vi "读取反控数据解析(子VI).vi"(6 "数据":string, 7 "命令编码CN":string) -> (0 "实时数据发送时间间隔/min":i32=1, 2 "设置超时时间/min":i32=1)   [LabVIEW 2016, in "数据传输系统.lvlib"]
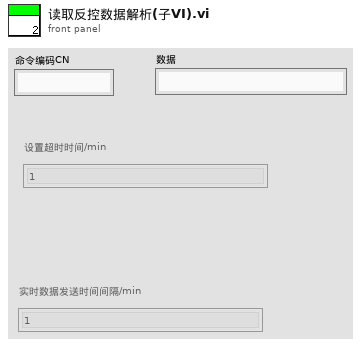
[diagram p1: front panel]
types:
  T1 = enum16{"初始化", "打开连接", "表格比对", "发送数据", "读取数据", "数据处理"}
  T2 = enum16{"CODMn", "CODCr", "氨氮", "总磷", "总氮", "数采仪"}
  T3 = cluster{"高锰酸盐":string, "化学需氧量":string, "氨氮":string, "总磷":string, "总氮":string, "数采仪":string, "高锰酸盐":bool, "化学需氧量":bool, "氨氮":bool, "总磷":bool, "总氮":bool, "数采仪":bool}
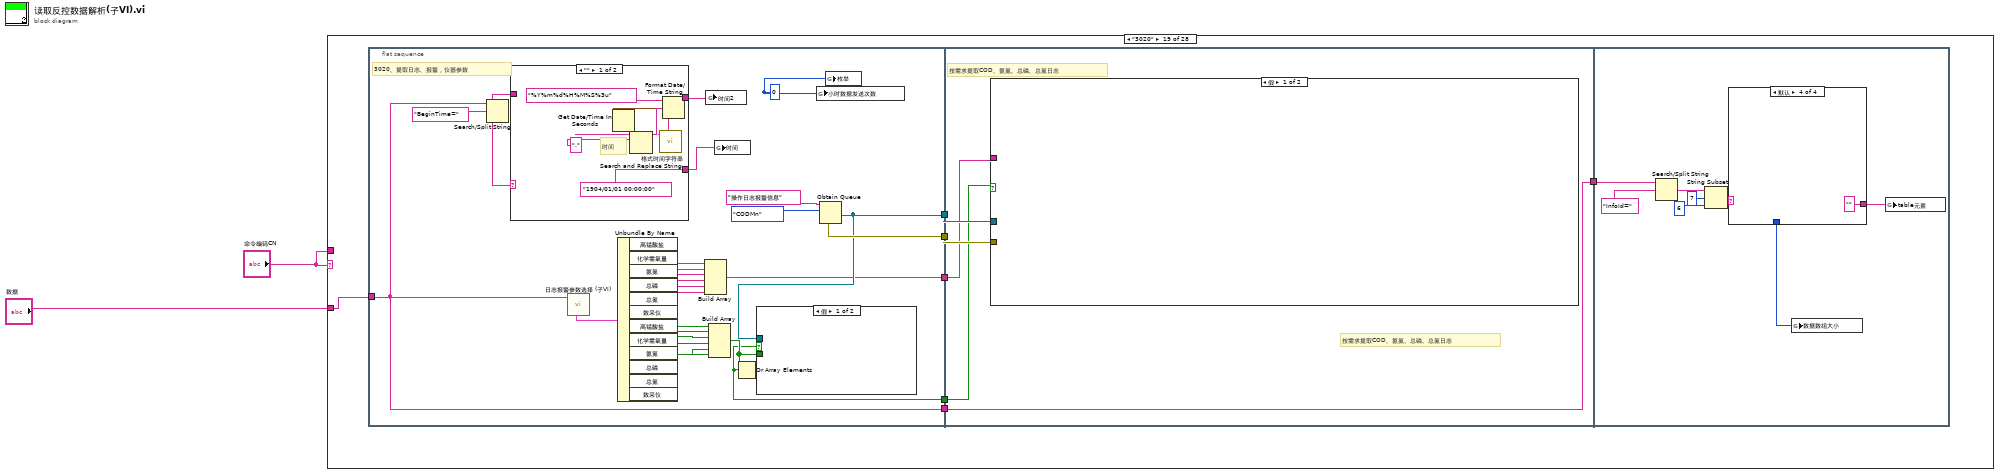
[diagram p0: block diagram]
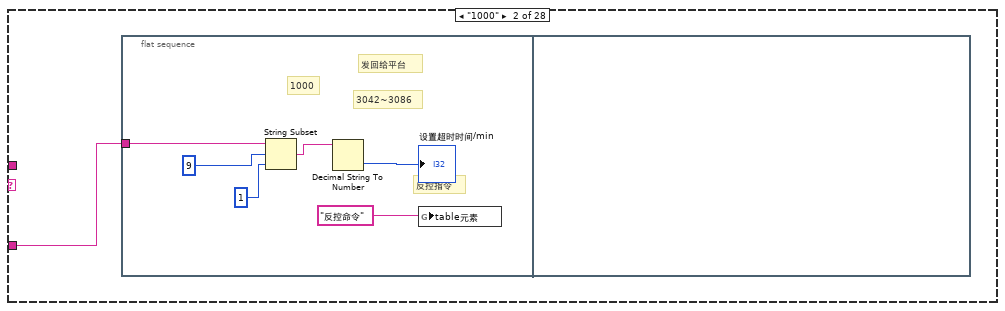
[diagram p3: hidden frame]
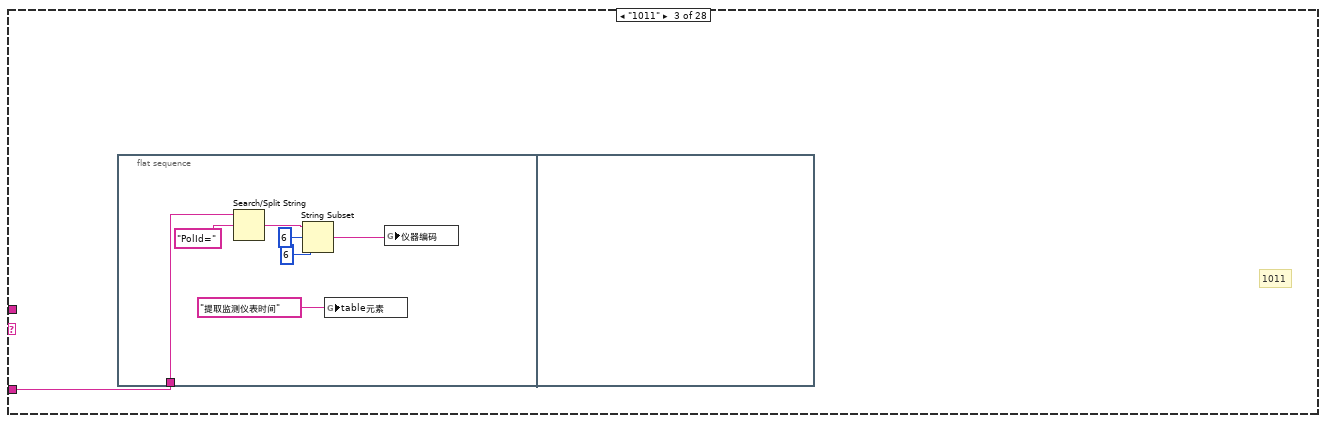
[diagram p4: hidden frame]
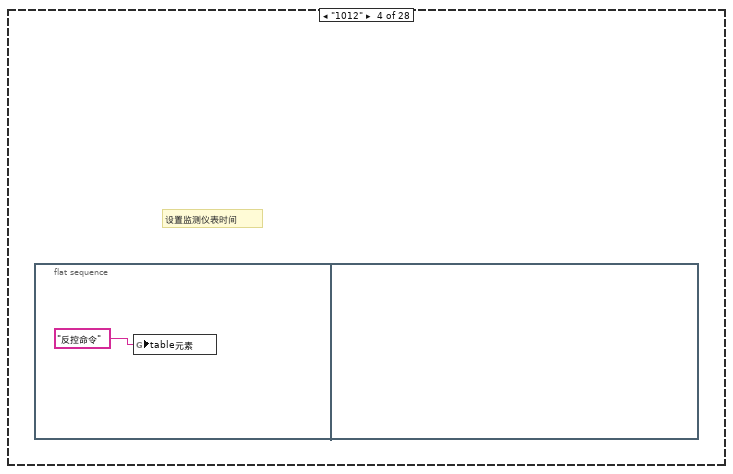
[diagram p5: hidden frame]
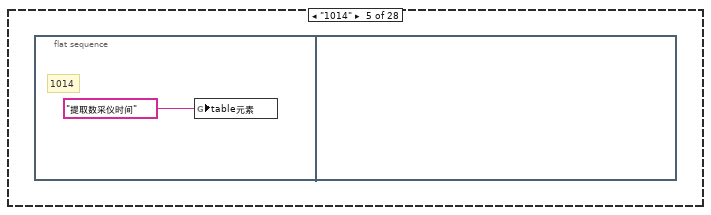
[diagram p6: hidden frame]
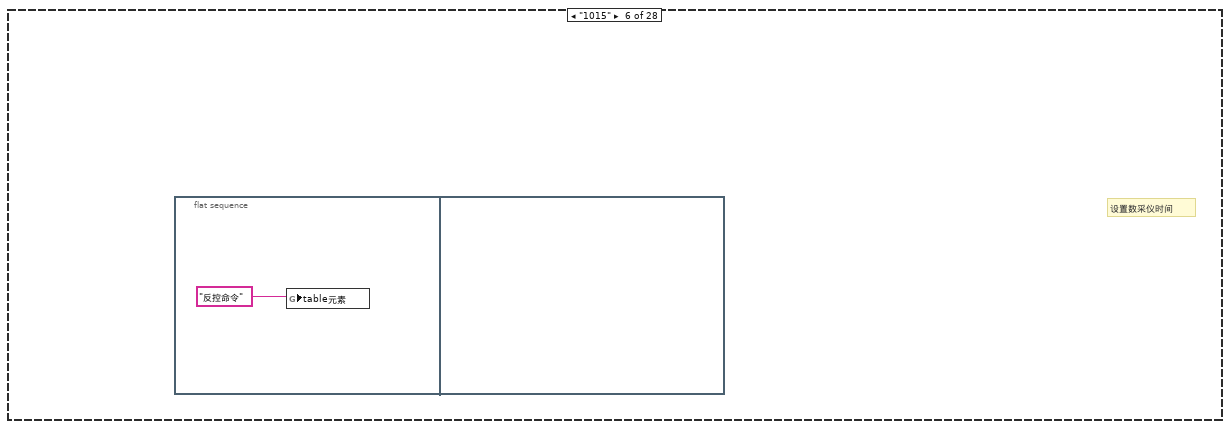
[diagram p7: hidden frame]
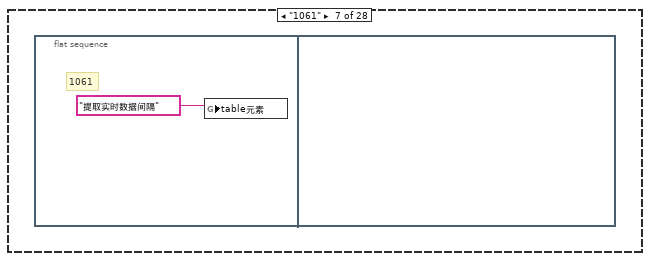
[diagram p8: hidden frame]
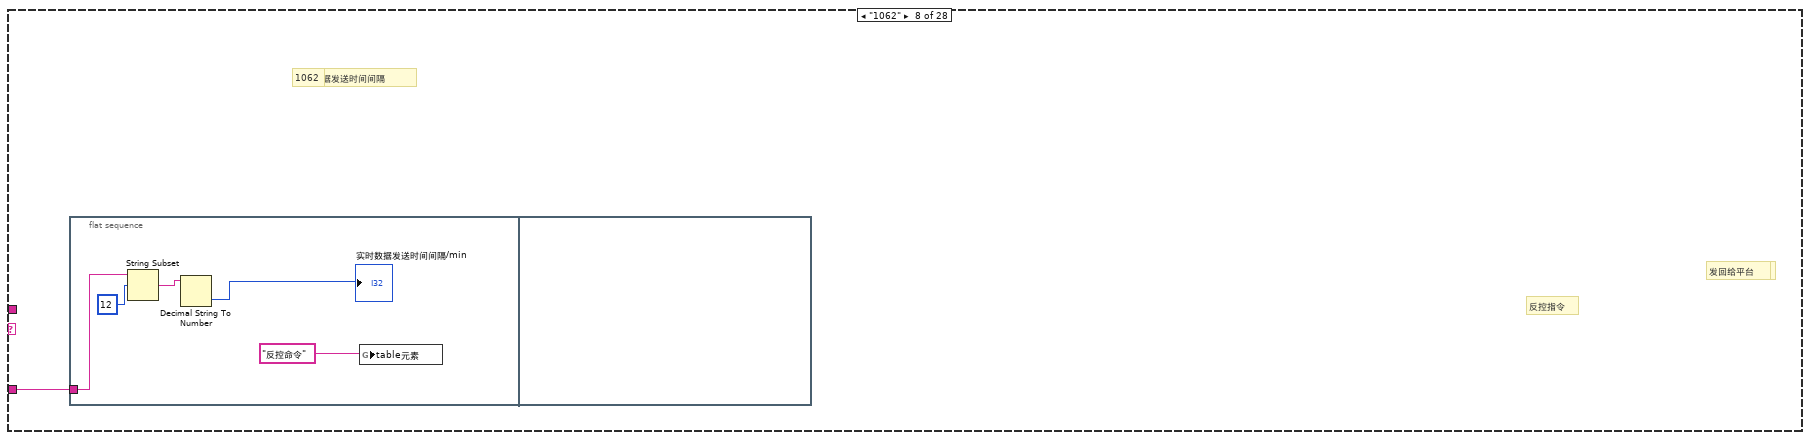
[diagram p9: hidden frame]
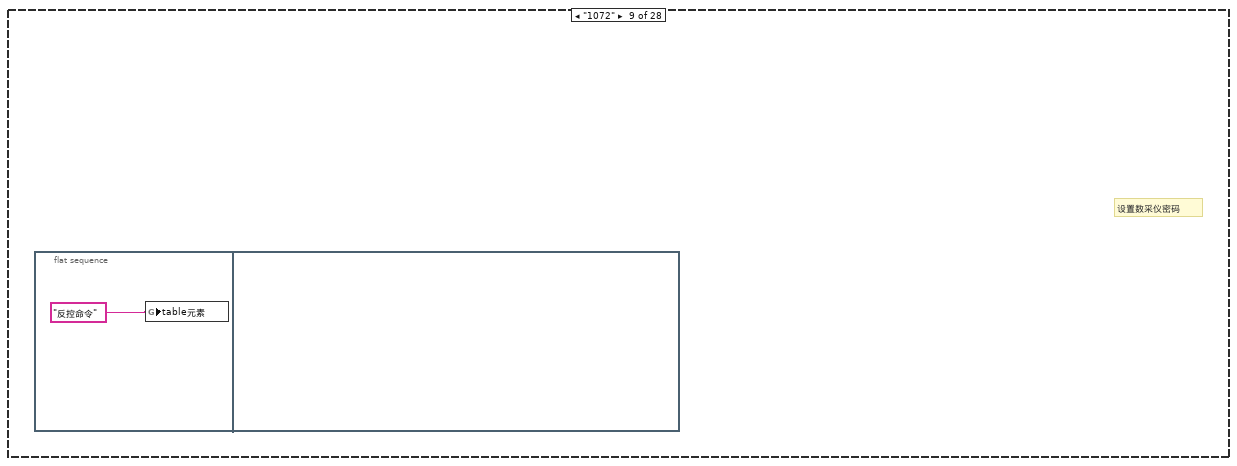
[diagram p10: hidden frame]
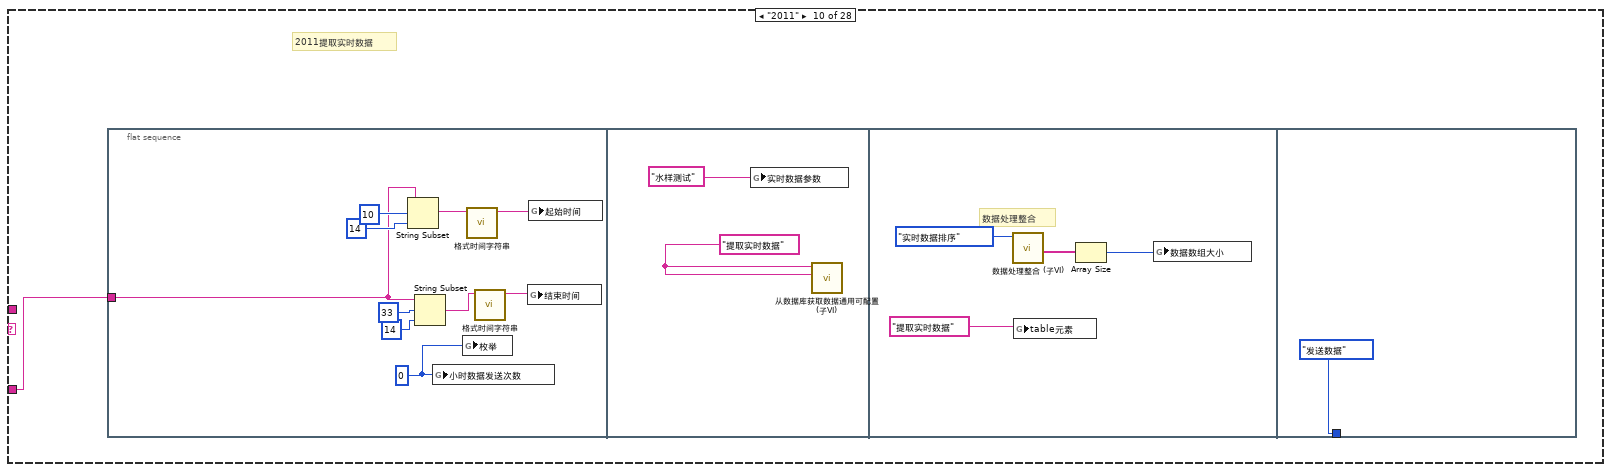
[diagram p11: hidden frame]
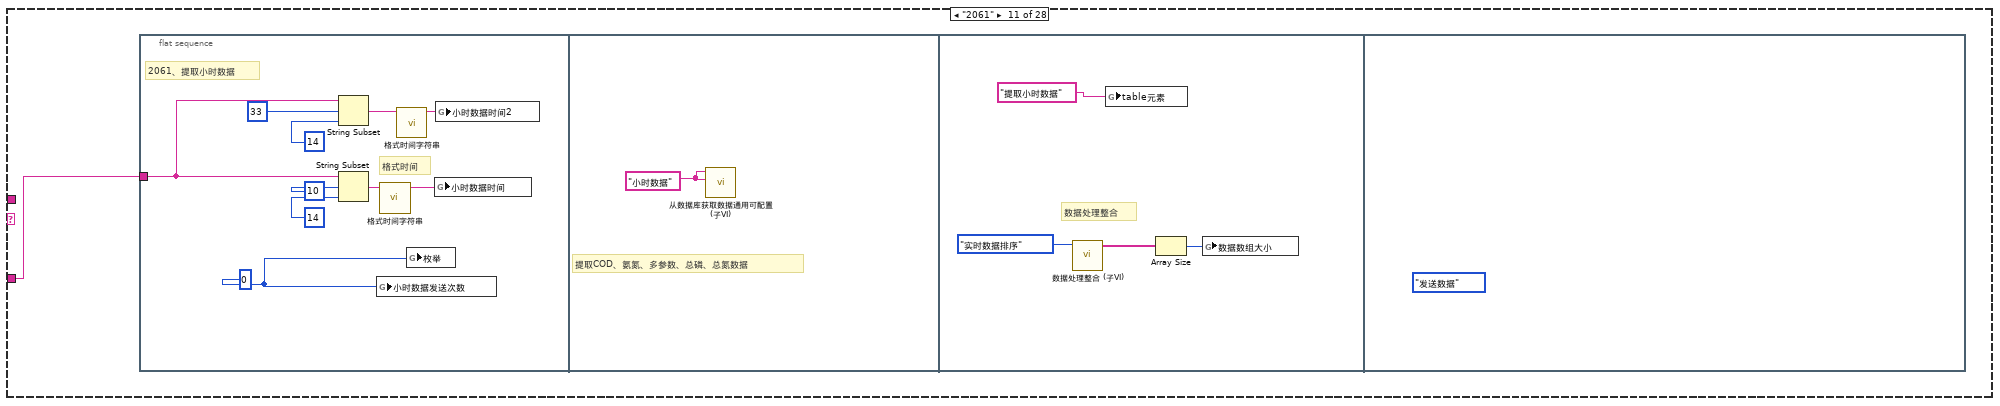
[diagram p12: hidden frame]
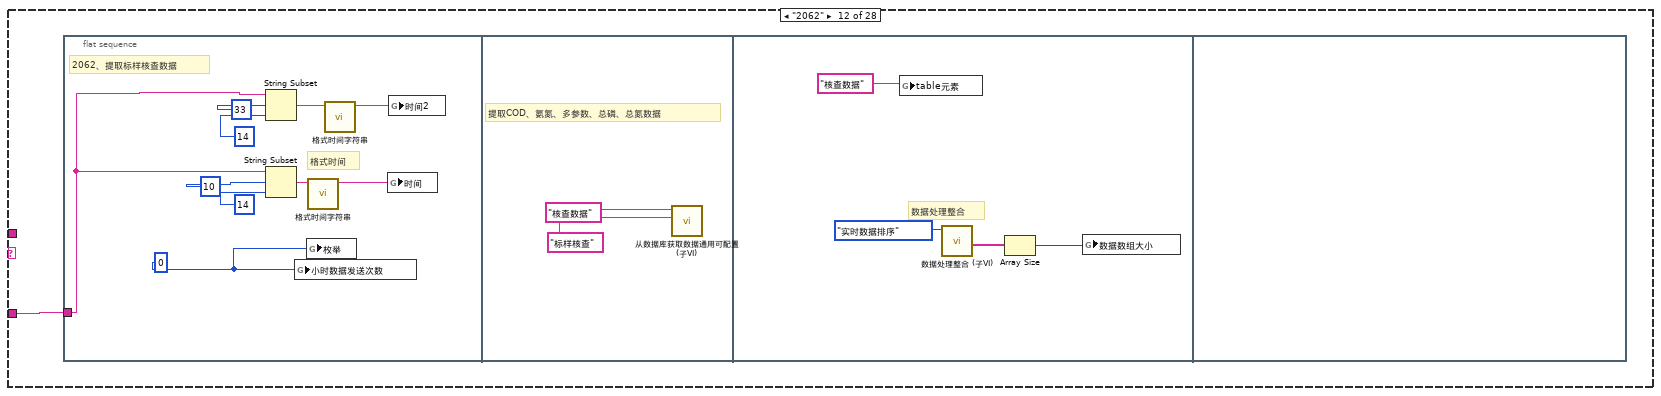
[diagram p13: hidden frame]
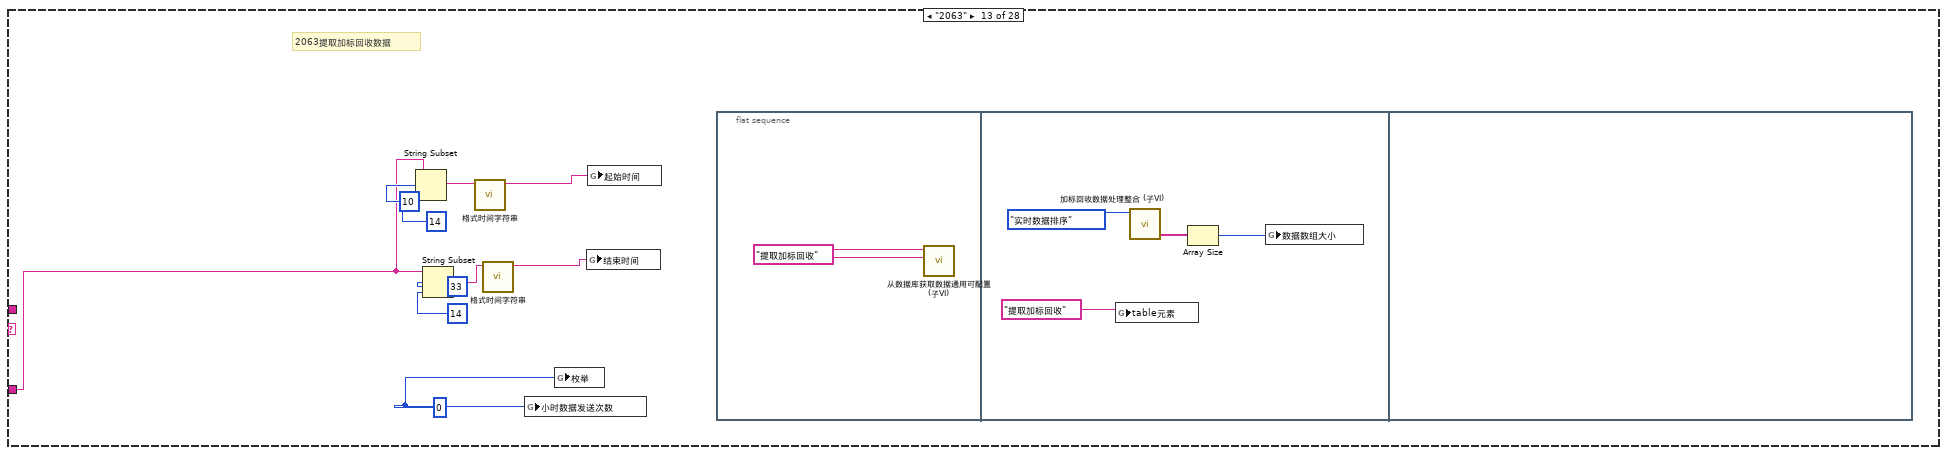
[diagram p14: hidden frame]
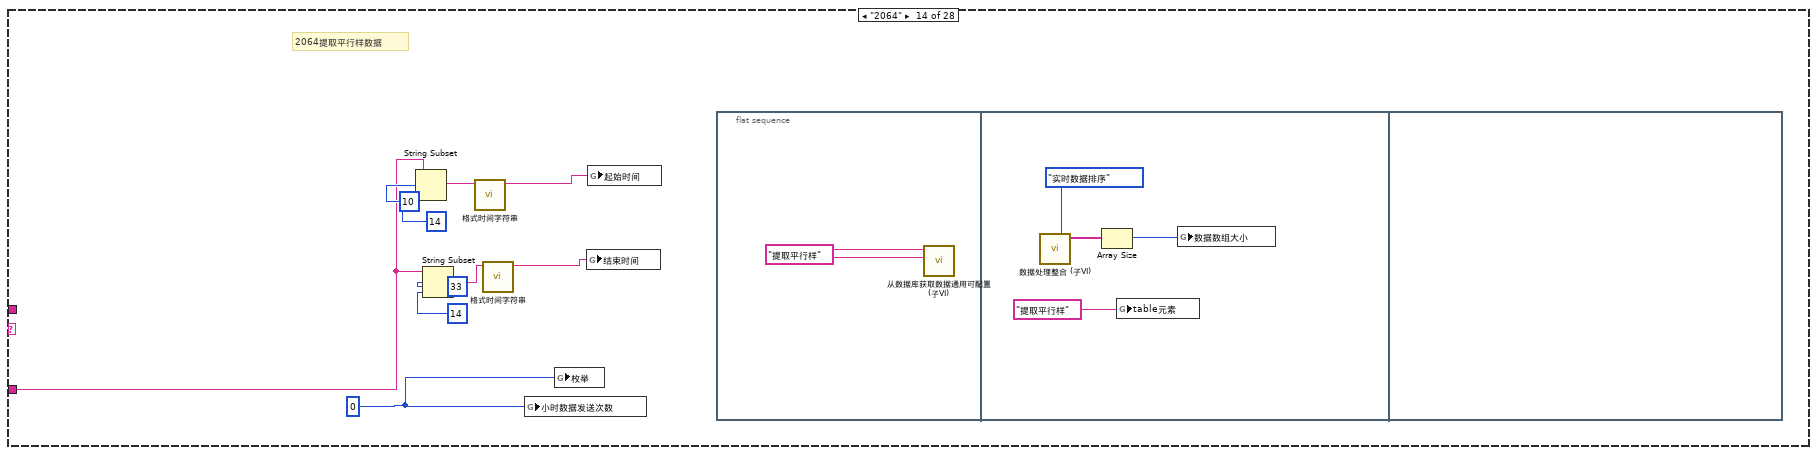
[diagram p15: hidden frame]
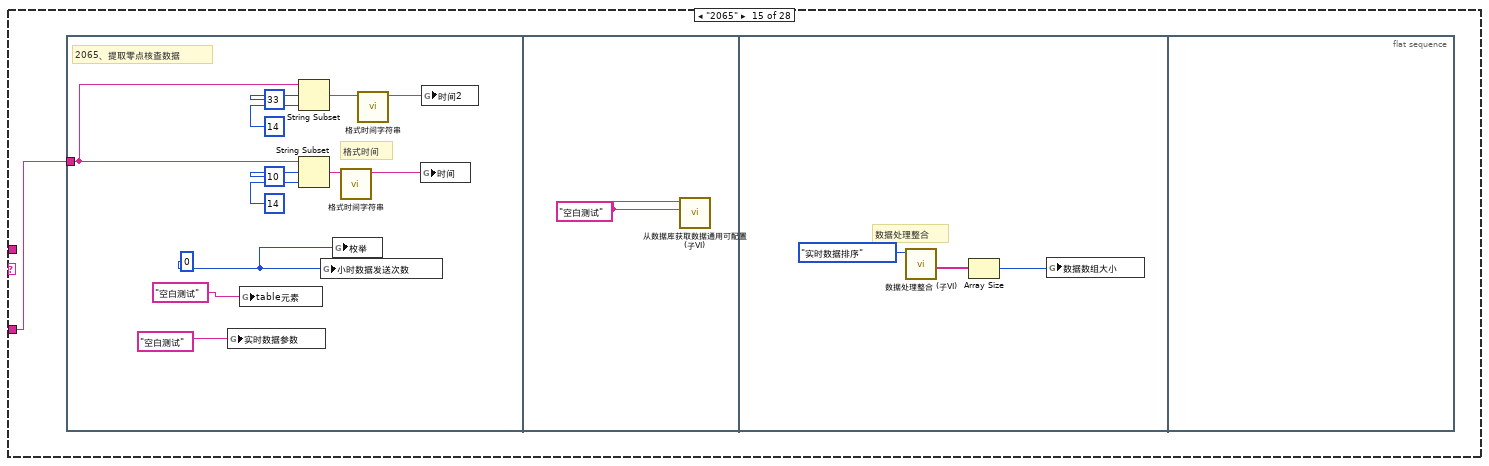
[diagram p16: hidden frame]
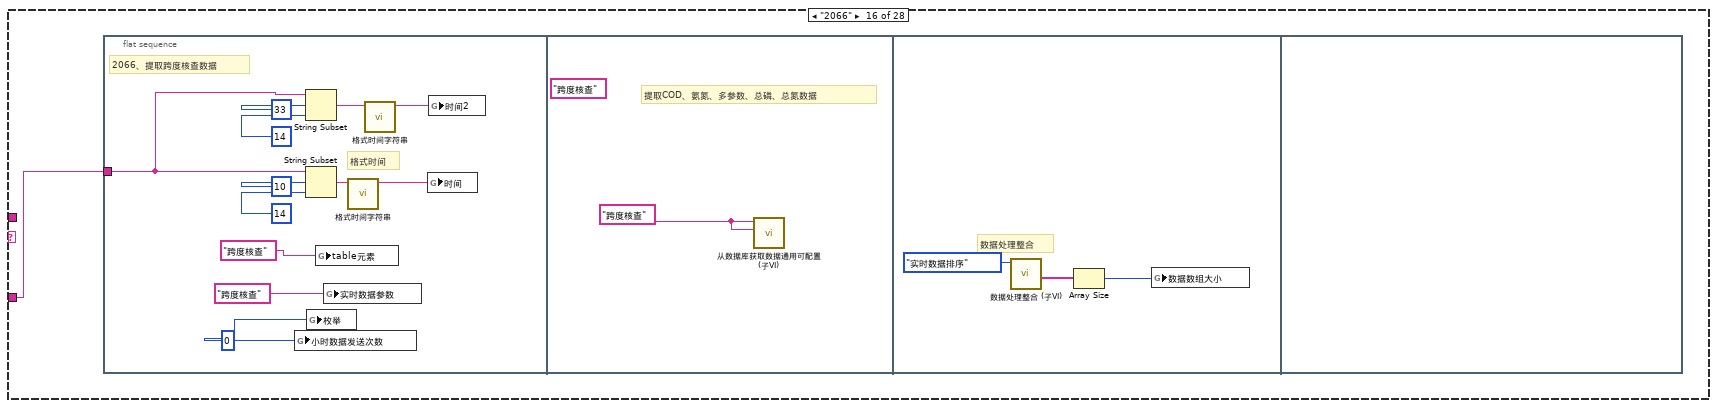
[diagram p17: hidden frame]
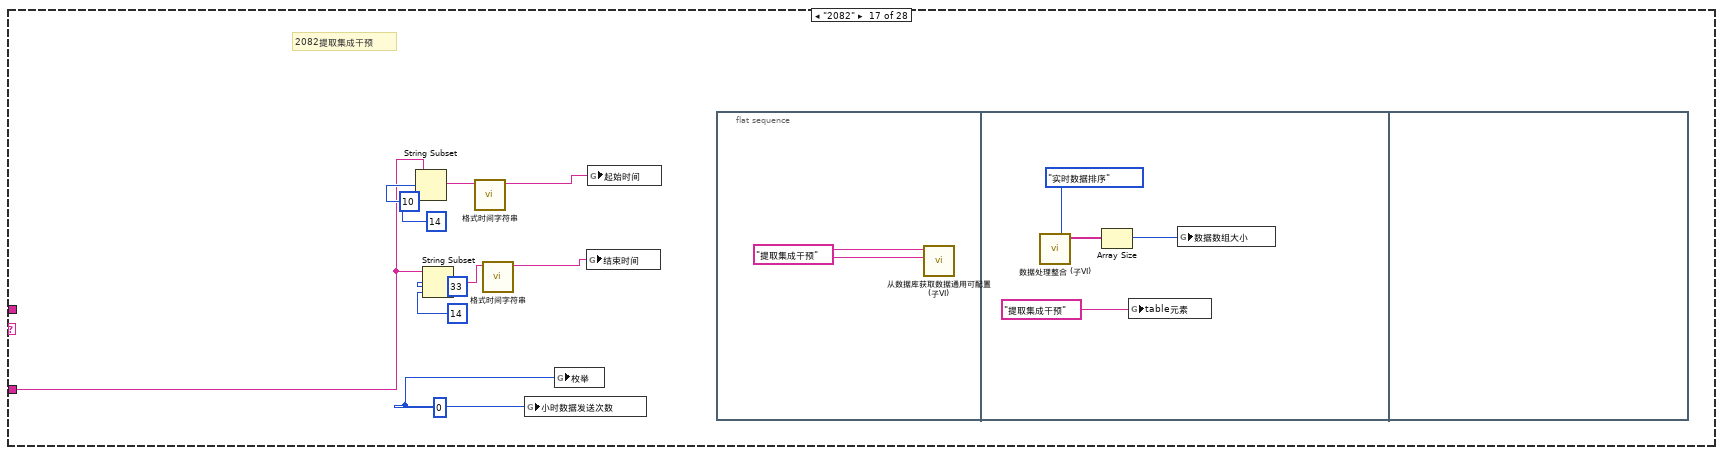
[diagram p18: hidden frame]
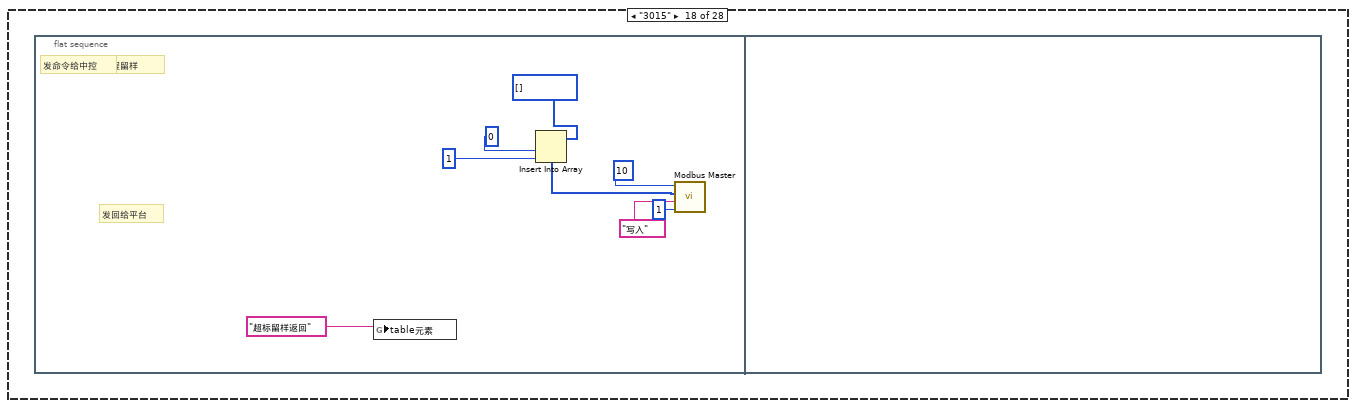
[diagram p19: hidden frame]
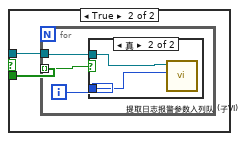
[diagram p20: hidden frame]
diagram:
  n1 = case shown="\"3020\"" "命令编码CN" {
    tunnel: "命令编码CN" -> [_ _ _ _ _ _ _ _ _ _ _ _ _ _ _ _ _ _ _ _ _ _ _ _ _ _ _ w353]
    tunnel: "数据" -> [_ w3 w10 _ _ _ _ w22 _ w29 w47 w63 w80 w95 w110 w127 w144 _ w169 _ _ _ w297 _ _ _ w337 w350]
    frame "", Default {
    }
    frame "1000" {
      n2 = flat-sequence {
        tunnel: w3 -> [w5]
        frame #0 {
          # "发回给平台"
          # "3042~3086"
          # "反控指令"
          # "1000"
          n3 = String Subset(string=w5, offset (0)=9 ("偏移量(0)"), length (rest)=1 ("长度（剩余）")) -> (substring=w7:string)
          n4 = Decimal String To Number(string=w7) -> (number=→"设置超时时间/min":i32)  [unwired: 2 in, 1 out]
          n5 = global write "全局1.vi" "table元素"("反控命令" ("新元素/子数组")) -> ()
        }
        frame #1 {
        }
      }
    }
    frame "1011" {
      # "1011"
      n6 = flat-sequence {
        tunnel: w10 -> [w12]
        frame #0 {
          n7 = Search/Split String(string=w12, search string/char (-)="PolId=" ("搜索字符串/字符(-)")) -> (match + rest of string=w16:string)  [unwired: 1 in, 2 out]
          n8 = String Subset(string=w16, offset (0)=6 ("偏移量(0)"), length (rest)=6 ("长度（剩余）")) -> (substring=w13:string)
          n9 = global write "全局1.vi" "table元素"("提取监测仪表时间") -> ()
          n10 = global write "全局 提取仪器参数.vi" "仪器编码"(w13) -> ()
        }
        frame #1 {
        }
      }
    }
    frame "1012" {
      # "设置监测仪表时间"
      n11 = flat-sequence {
        frame #0 {
          n12 = global write "全局1.vi" "table元素"("反控命令" ("新元素/子数组")) -> ()
        }
        frame #1 {
        }
      }
    }
    frame "1014" {
      n13 = flat-sequence {
        frame #0 {
          # "1014"
          n14 = global write "全局1.vi" "table元素"("提取数采仪时间") -> ()
        }
        frame #1 {
        }
      }
    }
    frame "1015" {
      # "设置数采仪时间"
      n15 = flat-sequence {
        frame #0 {
          n16 = global write "全局1.vi" "table元素"("反控命令" ("新元素/子数组")) -> ()
        }
        frame #1 {
        }
      }
    }
    frame "1061" {
      n17 = flat-sequence {
        frame #0 {
          # "1061"
          n18 = global write "全局1.vi" "table元素"("提取实时数据间隔") -> ()
        }
        frame #1 {
        }
      }
    }
    frame "1062" {
      # "发回给平台"
      # "反控指令"
      # "3042~3086"
      # "设置数据发送时间间隔"
      # "1062"
      n19 = flat-sequence {
        tunnel: w22 -> [w25]
        frame #0 {
          n20 = String Subset(string=w25, offset (0)=12 ("偏移量(0)")) -> (substring=w26:string)  [unwired: 1 in]
          n21 = Decimal String To Number(string=w26) -> (number=→"实时数据发送时间间隔/min":i32)  [unwired: 2 in, 1 out]
          n22 = global write "全局1.vi" "table元素"("反控命令" ("新元素/子数组")) -> ()
        }
        frame #1 {
        }
      }
    }
    frame "1072" {
      # "设置数采仪密码"
      n23 = flat-sequence {
        frame #0 {
          n24 = global write "全局1.vi" "table元素"("反控命令" ("新元素/子数组")) -> ()
        }
        frame #1 {
        }
      }
    }
    frame "2011" {
      # "2011提取实时数据"
      n25 = flat-sequence {
        tunnel: w29 -> [w30]
        tunnel: [T1."发送数据" ("元素")] -> _
        frame #0 {
          w35 = 0 ("数值")
          n26 = String Subset(string=w30, offset (0)=10 ("偏移量(0)"), length (rest)=14 ("长度（剩余）")) -> (substring=w38:string)
          n27 = String Subset(string=w30, offset (0)=33 ("偏移量(0)"), length (rest)=14 ("长度（剩余）")) -> (substring=w36:string)
          n28 = global write "全局 小时数据发送次数.vi" "小时数据发送次数"(w35) -> ()
          n29 = global write "全局1.vi" "枚举"(w35) -> ()
          n30 = call "格式时间字符串.vi"("字符串"=w38) -> ("连接的字符串"=w39:string)  [unwired: 10 in]
          n31 = call "格式时间字符串.vi"("字符串"=w36) -> ("连接的字符串"=w37:string)  [unwired: 10 in]
          n32 = global write "起始时间.vi" "结束时间"(w37) -> ()
          n33 = global write "起始时间.vi" "起始时间"(w39) -> ()
        }
        frame #1 {
          w40 = "提取实时数据" ("新元素/子数组")
          n34 = global write "全局 实时数据参数.vi" "实时数据参数"("水样测试") -> ()
          n35 = call "从数据库获取数据通用可配置(子VI).vi"("table输入"=w40, "列队名（唯一）"=w40) -> ()  [unwired: 8 in, 2 out]
        }
        frame #2 {
          # "数据处理整合"
          n36 = call "数据处理整合 (子VI).vi"("枚举"=enum16{"实时数据排序", "小时数据排序"}."实时数据排序") -> ("已排序的数组"=w44:string[])  [unwired: 10 in]
          n37 = global write "全局1.vi" "table元素"("提取实时数据" ("新元素/子数组")) -> ()
          n38 = Array Size(array=w44) -> (size(s)=w45:i32)
          n39 = global write "全局 数据数组大小.vi" "数据数组大小"(w45) -> ()
        }
        frame #3 {
        }
      }
    }
    frame "2061" {
      n40 = flat-sequence {
        tunnel: w47 -> [w48]
        frame #0 {
          w49 = 0 ("数值")
          # "格式时间"
          # "2061、提取小时数据"
          n41 = String Subset(string=w48, offset (0)=33 ("偏移量(0)"), length (rest)=14 ("长度（剩余）")) -> (substring=w51:string)
          n42 = String Subset(string=w48, offset (0)=10 ("偏移量(0)"), length (rest)=14 ("长度（剩余）")) -> (substring=w52:string)
          n43 = global write "全局 小时数据发送次数.vi" "小时数据发送次数"(w49) -> ()
          n44 = call "格式时间字符串.vi"("字符串"=w52) -> ("连接的字符串"=w53:string)  [unwired: 10 in]
          n45 = call "格式时间字符串.vi"("字符串"=w51) -> ("连接的字符串"=w50:string)  [unwired: 10 in]
          n46 = global write "全局1.vi" "枚举"(w49) -> ()
          n47 = global write "全局 水样时间.vi" "小时数据时间"(w53) -> ()
          n48 = global write "全局 时间2.vi" "小时数据时间2"(w50) -> ()
        }
        frame #1 {
          w58 = "小时数据" ("名称（未命名）")
          # "提取COD、氨氮、多参数、总磷、总氮数据"
          n49 = call "从数据库获取数据通用可配置(子VI).vi"("table输入"=w58, "列队名（唯一）"=w58) -> ()  [unwired: 8 in, 2 out]
        }
        frame #2 {
          # "数据处理整合"
          n50 = call "数据处理整合 (子VI).vi"("枚举"=enum16{"实时数据排序", "小时数据排序"}."实时数据排序") -> ("已排序的数组"=w62:string[])  [unwired: 10 in]
          n51 = global write "全局1.vi" "table元素"("提取小时数据" ("新元素/子数组")) -> ()
          n52 = Array Size(array=w62) -> (size(s)=w61:i32)
          n53 = global write "全局 数据数组大小.vi" "数据数组大小"(w61) -> ()
        }
        frame #3 {
          (unwired) T1."发送数据" ("元素")
        }
      }
    }
    frame "2062" {
      n54 = flat-sequence {
        tunnel: w63 -> [w64]
        frame #0 {
          w65 = 0 ("数值")
          # "格式时间"
          # "2062、提取标样核查数据"
          n55 = String Subset(string=w64, offset (0)=33 ("偏移量(0)"), length (rest)=14 ("长度（剩余）")) -> (substring=w67:string)
          n56 = String Subset(string=w64, offset (0)=10 ("偏移量(0)"), length (rest)=14 ("长度（剩余）")) -> (substring=w68:string)
          n57 = global write "全局 小时数据发送次数.vi" "小时数据发送次数"(w65) -> ()
          n58 = global write "全局1.vi" "枚举"(w65) -> ()
          n59 = call "格式时间字符串.vi"("字符串"=w68) -> ("连接的字符串"=w69:string)  [unwired: 10 in]
          n60 = call "格式时间字符串.vi"("字符串"=w67) -> ("连接的字符串"=w66:string)  [unwired: 10 in]
          n61 = global write "全局 水样时间.vi" "时间"(w69) -> ()
          n62 = global write "全局 时间2.vi" "时间2"(w66) -> ()
        }
        frame #1 {
          # "提取COD、氨氮、多参数、总磷、总氮数据"
          n63 = call "从数据库获取数据通用可配置(子VI).vi"("table输入"="标样核查" ("新元素/子数组"), "列队名（唯一）"="核查数据" ("新元素/子数组")) -> ()  [unwired: 8 in, 2 out]
        }
        frame #2 {
          # "数据处理整合"
          n64 = global write "全局1.vi" "table元素"("核查数据" ("新元素/子数组")) -> ()
          n65 = call "数据处理整合 (子VI).vi"("枚举"=enum16{"实时数据排序", "小时数据排序"}."实时数据排序") -> ("已排序的数组"=w78:string[])  [unwired: 10 in]
          n66 = Array Size(array=w78) -> (size(s)=w79:i32)
          n67 = global write "全局 数据数组大小.vi" "数据数组大小"(w79) -> ()
        }
        frame #3 {
        }
      }
    }
    frame "2063" {
      w85 = 0 ("数值")
      # "2063提取加标回收数据"
      n68 = String Subset(string=w80, offset (0)=10 ("偏移量(0)"), length (rest)=14 ("长度（剩余）")) -> (substring=w82:string)
      n69 = String Subset(string=w80, offset (0)=33 ("偏移量(0)"), length (rest)=14 ("长度（剩余）")) -> (substring=w84:string)
      n70 = call "格式时间字符串.vi"("字符串"=w82) -> ("连接的字符串"=w81:string)  [unwired: 10 in]
      n71 = call "格式时间字符串.vi"("字符串"=w84) -> ("连接的字符串"=w83:string)  [unwired: 10 in]
      n72 = global write "全局 小时数据发送次数.vi" "小时数据发送次数"(w85) -> ()
      n73 = global write "全局1.vi" "枚举"(w85) -> ()
      n74 = global write "起始时间.vi" "结束时间"(w83) -> ()
      n75 = global write "起始时间.vi" "起始时间"(w81) -> ()
      n76 = flat-sequence {
        frame #0 {
          w90 = "提取加标回收" ("新元素/子数组")
          n77 = call "从数据库获取数据通用可配置(子VI).vi"("table输入"=w90, "列队名（唯一）"=w90) -> ()  [unwired: 8 in, 2 out]
        }
        frame #1 {
          n78 = global write "全局1.vi" "table元素"("提取加标回收" ("新元素/子数组")) -> ()
          n79 = call "加标回收数据处理整合 (子VI).vi"("枚举"=enum16{"实时数据排序", "小时数据排序"}."实时数据排序") -> ("已排序的数组"=w92:string[])  [unwired: 10 in]
          n80 = Array Size(array=w92) -> (size(s)=w94:i32)
          n81 = global write "全局 数据数组大小.vi" "数据数组大小"(w94) -> ()
        }
        frame #2 {
        }
      }
    }
    frame "2064" {
      w100 = 0 ("数值")
      # "2064提取平行样数据"
      n82 = String Subset(string=w95, offset (0)=10 ("偏移量(0)"), length (rest)=14 ("长度（剩余）")) -> (substring=w97:string)
      n83 = String Subset(string=w95, offset (0)=33 ("偏移量(0)"), length (rest)=14 ("长度（剩余）")) -> (substring=w99:string)
      n84 = call "格式时间字符串.vi"("字符串"=w97) -> ("连接的字符串"=w96:string)  [unwired: 10 in]
      n85 = call "格式时间字符串.vi"("字符串"=w99) -> ("连接的字符串"=w98:string)  [unwired: 10 in]
      n86 = global write "全局 小时数据发送次数.vi" "小时数据发送次数"(w100) -> ()
      n87 = global write "全局1.vi" "枚举"(w100) -> ()
      n88 = global write "起始时间.vi" "结束时间"(w98) -> ()
      n89 = global write "起始时间.vi" "起始时间"(w96) -> ()
      n90 = flat-sequence {
        frame #0 {
          w105 = "提取平行样" ("新元素/子数组")
          n91 = call "从数据库获取数据通用可配置(子VI).vi"("table输入"=w105, "列队名（唯一）"=w105) -> ()  [unwired: 8 in, 2 out]
        }
        frame #1 {
          n92 = call "数据处理整合 (子VI).vi"("枚举"=enum16{"实时数据排序", "小时数据排序"}."实时数据排序") -> ("已排序的数组"=w109:string[])  [unwired: 10 in]
          n93 = Array Size(array=w109) -> (size(s)=w108:i32)
          n94 = global write "全局1.vi" "table元素"("提取平行样" ("新元素/子数组")) -> ()
          n95 = global write "全局 数据数组大小.vi" "数据数组大小"(w108) -> ()
        }
        frame #2 {
        }
      }
    }
    frame "2065" {
      n96 = flat-sequence {
        tunnel: w110 -> [w112]
        frame #0 {
          w113 = 0 ("数值")
          # "格式时间"
          # "2065、提取零点核查数据"
          n97 = global write "全局 实时数据参数.vi" "实时数据参数"("空白测试" ("新元素/子数组")) -> ()
          n98 = global write "全局1.vi" "table元素"("空白测试" ("新元素/子数组")) -> ()
          n99 = String Subset(string=w112, offset (0)=33 ("偏移量(0)"), length (rest)=14 ("长度（剩余）")) -> (substring=w116:string)
          n100 = String Subset(string=w112, offset (0)=10 ("偏移量(0)"), length (rest)=14 ("长度（剩余）")) -> (substring=w117:string)
          n101 = global write "全局 小时数据发送次数.vi" "小时数据发送次数"(w113) -> ()
          n102 = global write "全局1.vi" "枚举"(w113) -> ()
          n103 = call "格式时间字符串.vi"("字符串"=w117) -> ("连接的字符串"=w118:string)  [unwired: 10 in]
          n104 = call "格式时间字符串.vi"("字符串"=w116) -> ("连接的字符串"=w115:string)  [unwired: 10 in]
          n105 = global write "全局 水样时间.vi" "时间"(w118) -> ()
          n106 = global write "全局 时间2.vi" "时间2"(w115) -> ()
        }
        frame #1 {
          w123 = "空白测试" ("新元素/子数组")
          n107 = call "从数据库获取数据通用可配置(子VI).vi"("table输入"=w123, "列队名（唯一）"=w123) -> ()  [unwired: 8 in, 2 out]
        }
        frame #2 {
          # "数据处理整合"
          n108 = call "数据处理整合 (子VI).vi"("枚举"=enum16{"实时数据排序", "小时数据排序"}."实时数据排序") -> ("已排序的数组"=w125:string[])  [unwired: 10 in]
          n109 = Array Size(array=w125) -> (size(s)=w126:i32)
          n110 = global write "全局 数据数组大小.vi" "数据数组大小"(w126) -> ()
        }
        frame #3 {
        }
      }
    }
    frame "2066" {
      n111 = flat-sequence {
        tunnel: w127 -> [w129]
        frame #0 {
          w130 = 0 ("数值")
          # "格式时间"
          # "2066、提取跨度核查数据"
          n112 = global write "全局 小时数据发送次数.vi" "小时数据发送次数"(w130) -> ()
          n113 = String Subset(string=w129, offset (0)=33 ("偏移量(0)"), length (rest)=14 ("长度（剩余）")) -> (substring=w133:string)
          n114 = String Subset(string=w129, offset (0)=10 ("偏移量(0)"), length (rest)=14 ("长度（剩余）")) -> (substring=w134:string)
          n115 = global write "全局1.vi" "枚举"(w130) -> ()
          n116 = global write "全局1.vi" "table元素"("跨度核查" ("新元素/子数组")) -> ()
          n117 = global write "全局 实时数据参数.vi" "实时数据参数"("跨度核查" ("新元素/子数组")) -> ()
          n118 = call "格式时间字符串.vi"("字符串"=w134) -> ("连接的字符串"=w135:string)  [unwired: 10 in]
          n119 = call "格式时间字符串.vi"("字符串"=w133) -> ("连接的字符串"=w132:string)  [unwired: 10 in]
          n120 = global write "全局 水样时间.vi" "时间"(w135) -> ()
          n121 = global write "全局 时间2.vi" "时间2"(w132) -> ()
        }
        frame #1 {
          w140 = "跨度核查" ("新元素/子数组")
          (unwired) "跨度核查" ("名称（未命名）")
          # "提取COD、氨氮、多参数、总磷、总氮数据"
          n122 = call "从数据库获取数据通用可配置(子VI).vi"("table输入"=w140, "列队名（唯一）"=w140) -> ()  [unwired: 8 in, 2 out]
        }
        frame #2 {
          # "数据处理整合"
          n123 = call "数据处理整合 (子VI).vi"("枚举"=enum16{"实时数据排序", "小时数据排序"}."实时数据排序") -> ("已排序的数组"=w143:string[])  [unwired: 10 in]
          n124 = Array Size(array=w143) -> (size(s)=w142:i32)
          n125 = global write "全局 数据数组大小.vi" "数据数组大小"(w142) -> ()
        }
        frame #3 {
        }
      }
    }
    frame "2082" {
      w149 = 0 ("数值")
      # "2082提取集成干预"
      n126 = String Subset(string=w144, offset (0)=10 ("偏移量(0)"), length (rest)=14 ("长度（剩余）")) -> (substring=w146:string)
      n127 = String Subset(string=w144, offset (0)=33 ("偏移量(0)"), length (rest)=14 ("长度（剩余）")) -> (substring=w148:string)
      n128 = call "格式时间字符串.vi"("字符串"=w146) -> ("连接的字符串"=w145:string)  [unwired: 10 in]
      n129 = call "格式时间字符串.vi"("字符串"=w148) -> ("连接的字符串"=w147:string)  [unwired: 10 in]
      n130 = global write "全局 小时数据发送次数.vi" "小时数据发送次数"(w149) -> ()
      n131 = global write "全局1.vi" "枚举"(w149) -> ()
      n132 = global write "起始时间.vi" "结束时间"(w147) -> ()
      n133 = global write "起始时间.vi" "起始时间"(w145) -> ()
      n134 = flat-sequence {
        frame #0 {
          w154 = "提取集成干预" ("新元素/子数组")
          n135 = call "从数据库获取数据通用可配置(子VI).vi"("table输入"=w154, "列队名（唯一）"=w154) -> ()  [unwired: 8 in, 2 out]
        }
        frame #1 {
          n136 = call "数据处理整合 (子VI).vi"("枚举"=enum16{"实时数据排序", "小时数据排序"}."实时数据排序") -> ("已排序的数组"=w158:string[])  [unwired: 10 in]
          n137 = Array Size(array=w158) -> (size(s)=w157:i32)
          n138 = global write "全局1.vi" "table元素"("提取集成干预" ("新元素/子数组")) -> ()
          n139 = global write "全局 数据数组大小.vi" "数据数组大小"(w157) -> ()
        }
        frame #2 {
        }
      }
    }
    frame "3015" {
      n140 = flat-sequence {
        frame #0 {
          # "发命令给中控"
          # "发回给平台"
          # "3015、手动远程留样"
          n141 = global write "全局1.vi" "table元素"("超标留样返回" ("新元素/子数组")) -> ()
          n142 = Insert Into Array(array=u16[] [] ("holding register values"), index=0 ("索引"), new element=u16 1 ("新元素/子数组")) -> (w162:u16[])
          n143 = call "Modbus Master.vi"("Unit ID"=u8 1, "读取写入选择"="写入", "holding register values"=w162, "starting address"=u16 10) -> ()  [unwired: 6 in, 2 out]
        }
        frame #1 {
        }
      }
    }
    frame "3020" {
      n144 = flat-sequence {
        tunnel: [w178] -> w173
        tunnel: [w179] -> w172
        tunnel: [w177] -> w171
        tunnel: [w175] -> w170
        tunnel: w169 -> [w174]
        tunnel: [w174] -> w167
        tunnel: w173 -> [w227]
        tunnel: w172 -> [w226]
        tunnel: w171 -> [w225]
        tunnel: w170 -> [w224]
        tunnel: [w223] -> w168
        tunnel: w167 -> [w223]
        tunnel: w168 -> [w275]
        frame #0 {
          w197 = 0 ("数值")
          # "3020、提取日志、报警，仪器参数"
          n145 = Search/Split String(string=w174, search string/char (-)="BeginTime=" ("搜索字符串")) -> (match + rest of string=w196:string)  [unwired: 1 in, 2 out]
          n146 = case shown="\"\"" w196 {
            tunnel: ["1904/01/01 00:00:00" w220] -> w199
            tunnel: w196 -> [_ w214]
            tunnel: [w207 w215] -> w195
            frame "" {
              # "时间"
              n147 = Get Date/Time In Seconds() -> (seconds since 1Jan1904=w208:timestamp)
              n148 = Format Date/Time String(time format string (%c)="%Y%m%d%H%M%S%3u" ("时间格式字符串(%c)"), seconds (now)=w208) -> (date/time string=w212:string)  [unwired: 1 in]
              n149 = Search and Replace String(input string=w212, search string="." ("搜索字符串")) -> (result string=w211:string)  [unwired: 6 in, 3 out]
              n150 = call "格式时间字符串.vi"("字符串"=w211) -> ("连接的字符串"=w207:string)  [unwired: 10 in]
            }
            frame "真", Default {
              # "格式时间"
              n151 = String Subset(string=w214, offset (0)=33 ("偏移量(0)"), length (rest)=14 ("长度（剩余）")) -> (substring=w218:string)
              n152 = String Subset(string=w214, offset (0)=10 ("偏移量(0)"), length (rest)=14 ("长度（剩余）")) -> (substring=w219:string)
              n153 = call "格式时间字符串.vi"("字符串"=w218) -> ("连接的字符串"=w215:string)  [unwired: 10 in]
              n154 = call "格式时间字符串.vi"("字符串"=w219) -> ("连接的字符串"=w220:string)  [unwired: 10 in]
            }
          }
          n155 = call "日志报警参数选择 (子VI).vi"("String输入"=w174) -> ("输出簇"=w182:T3)  [unwired: 9 in, 1 out]
          n156 = Unbundle By Name(w182) -> ("高锰酸盐"=w189:string, "化学需氧量"=w190:string, "氨氮"=w191:string, "总磷"=w192:string, "总氮"=w193:string, "数采仪"=w194:string, "高锰酸盐"=w183:bool, "化学需氧量"=w184:bool, "氨氮"=w185:bool, "总磷"=w186:bool, "总氮"=w187:bool, "数采仪"=w188:bool)
          n157 = Build Array(w189, w190, w191, w192, w193, w194) -> (w177:string[])
          n158 = global write "全局 时间2.vi" "时间2"(w195) -> ()
          n159 = Build Array(w183, w184, w185, w186, w187, w188) -> (w176:bool[])
          n160 = global write "全局 水样时间.vi" "时间"(w199) -> ()
          n161 = Or Array Elements(Boolean array=w176) -> (logical OR=w175:bool)
          n162 = global write "全局 小时数据发送次数.vi" "小时数据发送次数"(w197) -> ()
          n163 = Obtain Queue(name (unnamed)="操作日志报警信息" ("名称（未命名）"), element data type=T2."CODMn") -> (queue out=w178:refnum<queue>, error out=w179:errorcluster)  [unwired: 3 in, 1 out]
          n164 = case shown="假" w175 {
            tunnel: w178 -> [_ w201]
            tunnel: w176 -> [_ w200]
            frame False {
            }
            frame True {
              n165 = for {
                tunnel: w200 -> [w203] mode=indexing
                tunnel: w201 -> [w202]
                i -> [w204]
                n166 = case shown="真" w203 {
                  tunnel: w204 -> [_ w206]
                  tunnel: w202 -> [_ w205]
                  frame False {
                  }
                  frame True {
                    n167 = call "提取日志报警参数入列队 (子VI).vi"("枚举"=w206, "queue in"=w205) -> ()  [unwired: 10 in]
                  }
                }
              }
            }
          }
          n168 = global write "全局1.vi" "枚举"(w197) -> ()
        }
        frame #1 {
          # "按需求提取COD、氨氮、总磷、总氮日志"
          # "按需求提取COD、氨氮、总磷、总氮日志"
          n169 = case shown="假" w224 {
            tunnel: w226 -> [_ w230]
            tunnel: w227 -> [_ w229]
            tunnel: w225 -> [_ w228]
            frame False {
            }
            frame True {
              n170 = while {
                shift-right: [w244] -> _
                shift-left: w229 -> [w245]
                tunnel: w230 -> [w243]
                tunnel: w228 -> [w238]
                stop <- w240 stop-if-true
                n171 = Dequeue Element(queue=w245, error in (no error)=w243) -> (queue out=w242:refnum<queue>, element=w237:T2)  [unwired: 1 in, 2 out]
                n172 = Index Array(array=w238) -> (element #1=w236:string, element #2=w235:string, element #3=w234:string, element #4=w233:string, element #5=w232:string, element #6=w231:string)  [unwired: 6 in]
                n173 = case shown="\"CODMn\"" w237 {
                  tunnel: w242 -> [w250 _ w259 w264 w268 w273]
                  tunnel: [w250 _ w259 w264 w268 w273] -> w244
                  tunnel: w236 -> [w247 _ _ _ _ _]
                  tunnel: w235 -> [_ w252 _ _ _ _]
                  tunnel: w234 -> [_ _ w256 _ _ _]
                  tunnel: w233 -> [_ _ _ w261 _ _]
                  tunnel: w232 -> [_ _ _ _ w266 _]
                  tunnel: w231 -> [_ _ _ _ _ w270]
                  frame "CODMn" {
                    w246 = string[][] [] ("氨氮")
                    n174 = call "数据表比对.vi"("仪器日志参数"="CODMn" ("元素"), "table输入"=w247) -> ("待发送数据"=w248:string[][])  [unwired: 7 in, 2 out]
                    n175 = global write "全局 所有参数.vi" "CODMn"(w248) -> ()
                    n176 = global write "全局 所有参数.vi" "总氮"(w246) -> ()
                    n177 = global write "全局 所有参数.vi" "CODCr"(w246) -> ()
                    n178 = global write "全局 所有参数.vi" "总磷"(w246) -> ()
                    n179 = global write "全局 所有参数.vi" "氨氮"(w246) -> ()
                  }
                  frame "CODCr" {
                    w251 = string[][] [] ("氨氮")
                    n180 = call "数据表比对.vi"("仪器日志参数"="CODCr" ("元素"), "table输入"=w252) -> ("待发送数据"=w253:string[][])  [unwired: 7 in, 2 out]
                    n181 = global write "全局 所有参数.vi" "CODCr"(w253) -> ()
                    n182 = global write "全局 所有参数.vi" "CODMn"(w251) -> ()
                    n183 = global write "全局 所有参数.vi" "总氮"(w251) -> ()
                    n184 = global write "全局 所有参数.vi" "总磷"(w251) -> ()
                    n185 = global write "全局 所有参数.vi" "氨氮"(w251) -> ()
                  }
                  frame "氨氮" {
                    w255 = string[][] [] ("氨氮")
                    n186 = call "数据表比对.vi"("仪器日志参数"="氨氮" ("元素"), "table输入"=w256) -> ("待发送数据"=w257:string[][])  [unwired: 7 in, 2 out]
                    n187 = global write "全局 所有参数.vi" "氨氮"(w257) -> ()
                    n188 = global write "全局 所有参数.vi" "CODMn"(w255) -> ()
                    n189 = global write "全局 所有参数.vi" "总氮"(w255) -> ()
                    n190 = global write "全局 所有参数.vi" "CODCr"(w255) -> ()
                    n191 = global write "全局 所有参数.vi" "总磷"(w255) -> ()
                  }
                  frame "总磷" {
                    w260 = string[][] [] ("氨氮")
                    n192 = call "数据表比对.vi"("仪器日志参数"="总磷" ("元素"), "table输入"=w261) -> ("待发送数据"=w262:string[][])  [unwired: 7 in, 2 out]
                    n193 = global write "全局 所有参数.vi" "总磷"(w262) -> ()
                    n194 = global write "全局 所有参数.vi" "CODMn"(w260) -> ()
                    n195 = global write "全局 所有参数.vi" "总氮"(w260) -> ()
                    n196 = global write "全局 所有参数.vi" "CODCr"(w260) -> ()
                    n197 = global write "全局 所有参数.vi" "氨氮"(w260) -> ()
                  }
                  frame "总氮" {
                    w265 = string[][] [] ("氨氮")
                    n198 = call "数据表比对.vi"("仪器日志参数"="总氮" ("元素"), "table输入"=w266) -> ("待发送数据"=w267:string[][])  [unwired: 7 in, 2 out]
                    n199 = global write "全局 所有参数.vi" "总氮"(w267) -> ()
                    n200 = global write "全局 所有参数.vi" "CODMn"(w265) -> ()
                    n201 = global write "全局 所有参数.vi" "氨氮"(w265) -> ()
                    n202 = global write "全局 所有参数.vi" "CODCr"(w265) -> ()
                    n203 = global write "全局 所有参数.vi" "总磷"(w265) -> ()
                  }
                  frame "数采仪" {
                    n204 = call "数据表比对.vi"("仪器日志参数"="系统" ("元素"), "table输入"=w270) -> ("待发送数据"=w271:string[][])  [unwired: 7 in, 2 out]
                    n205 = global write "全局 所有参数.vi" "DO"(w271) -> ()
                  }
                }
                n206 = Get Queue Status(queue=w242) -> (# elements in queue=w241:i32)  [unwired: 2 in, 7 out]
                n207 = Wait (ms)(milliseconds to wait=u32 300 ("等待时间（毫秒）")) -> ()  [unwired: 1 out]
                n208 = Equal To 0?(x=w241) -> (x = 0?=w240:bool)
              }
            }
          }
        }
        frame #2 {
          n209 = Search/Split String(string=w275, search string/char (-)="InfoId=" ("搜索字符串/字符(-)")) -> (match + rest of string=w280:string)  [unwired: 1 in, 2 out]
          n210 = String Subset(string=w280, offset (0)=7 ("偏移量(0)"), length (rest)=6 ("长度（剩余）")) -> (substring=w277:string)
          n211 = case shown="默认" w277 {
            selector: w277 -> [_ w286 _ _]
            tunnel: ["操作日志" ("名称（未命名）") "提取仪器参数" ("名称（未命名）") "报警信息" ("名称（未命名）") "" ("名称（未命名）")] -> w274
            tunnel: [w282 1 ("数据数组大小") w289 _] -> w276
            frame "i11001", "i21001" {
              # "数据处理整合"
              # "i11001日志"
              n212 = call "数据处理整合 (子VI).vi"("枚举"=enum16{"实时数据排序", "小时数据排序"}."实时数据排序") -> ("已排序的数组"=w283:string[])  [unwired: 10 in]
              n213 = Array Size(array=w283) -> (size(s)=w282:i32)
            }
            frame "i13001", "i13002", "i13003", "i13004", "i13005", "i13006", "i13007", "i13008", "i13009", "i13010", "i13011", "i13012", "i13013" {
              n214 = global write "全局 提取仪器参数.vi" "参数编码"(w286) -> ()
              n215 = call "数据处理直接插入整合 (子VI).vi"() -> ()  [unwired: 12 in]
            }
            frame "i12001" {
              # "数据处理整合"
              # "i12001状态"
              n216 = call "数据处理整合 (子VI).vi"("枚举"=enum16{"实时数据排序", "小时数据排序"}."实时数据排序") -> ("已排序的数组"=w290:string[])  [unwired: 10 in]
              n217 = Array Size(array=w290) -> (size(s)=w289:i32)
            }
            frame Default {
            }
          }
          n218 = global write "全局 数据数组大小.vi" "数据数组大小"(w276) -> ()
          n219 = global write "全局1.vi" "table元素"(w274) -> ()
        }
      }
    }
    frame "3021" {
      n220 = flat-sequence {
        frame #0 {
          # "设置仪表参数"
          n221 = global write "全局1.vi" "table元素"("反控命令" ("新元素/子数组")) -> ()
        }
        frame #1 {
        }
      }
    }
    frame "3040" {
      # "提取现场系统信息（3040）"
      n222 = flat-sequence {
        frame #0 {
          n223 = global write "全局1.vi" "table元素"("提取现场系统信息" ("新元素/子数组")) -> ()
        }
        frame #1 {
        }
      }
    }
    frame "3041" {
      # "提取现场经纬度及环境信息（3041）"
      n224 = flat-sequence {
        frame #0 {
          n225 = call "获取环境参数 (子VI).vi"() -> ()  [unwired: 12 in]
          n226 = global write "全局1.vi" "table元素"("提取经纬度环境信息" ("新元素/子数组")) -> ()
        }
        frame #1 {
        }
      }
    }
    frame "3042" {
      n227 = flat-sequence {
        tunnel: w297 -> [w299]
        frame #0 {
          # "反控指令"
          # "反控指令\n切换运行模式"
          # "发命令给中控"
          # "0维护，1常规，2应急，3质控"
          n228 = Search/Split String(string=w299, search string/char (-)="RunMode" ("搜索字符串/字符(-)")) -> (match + rest of string=w310:string)  [unwired: 1 in, 2 out]
          n229 = String Subset(string=w310, offset (0)=8 ("偏移量(0)"), length (rest)=1 ("长度（剩余）")) -> (substring=w307:string)
          n230 = case shown="\"2\"" w307 {
            tunnel: [u16 0 ("新元素/子数组") u16 1 ("新元素/子数组") u16 2 ("新元素/子数组") u16 3 ("新元素/子数组")] -> w303
            frame "0", Default {
            }
            frame "1" {
            }
            frame "2" {
            }
            frame "3" {
            }
          }
          n231 = global write "全局1.vi" "table元素"("反控命令" ("新元素/子数组")) -> ()
          n232 = Insert Into Array(array=u16[] [] ("holding register values"), index=0 ("索引"), new element=w303) -> (w304:u16[])
          n233 = call "Modbus Master.vi"("Unit ID"=u8 1, "读取写入选择"="写入", "holding register values"=w304, "starting address"=u16 0) -> ()  [unwired: 6 in, 2 out]
        }
        frame #1 {
        }
      }
    }
    frame "3043" {
      # "远程重启数采仪"
      n234 = flat-sequence {
        frame #0 {
          n235 = global write "全局1.vi" "table元素"("反控命令" ("新元素/子数组")) -> ()
        }
        frame #1 {
        }
      }
    }
    frame "3044" {
      n236 = flat-sequence {
        frame #0 {
          # "反控指令"
          # "发命令给中控"
          n237 = call "Modbus Master.vi"("Unit ID"=u8 1, "读取写入选择"="写入", "holding register values"=u16[] [1], "starting address"=u16 2) -> ()  [unwired: 6 in, 2 out]
        }
        frame #1 {
          # "反控指令\n单次测量"
          n238 = Wait (ms)(milliseconds to wait=u32 500 ("等待时间（毫秒）")) -> ()  [unwired: 1 out]
        }
        frame #2 {
          n239 = global write "全局1.vi" "table元素"("反控命令" ("新元素/子数组")) -> ()
          n240 = call "Modbus Master.vi"("Unit ID"=u8 1, "读取写入选择"="写入", "holding register values"=u16[] [0], "starting address"=u16 2) -> ()  [unwired: 6 in, 2 out]
        }
        frame #3 {
        }
      }
    }
    frame "3045", "3046" {
      n241 = flat-sequence {
        frame #0 {
          # "发命令给中控"
          n242 = call "Modbus Master.vi"("Unit ID"=u8 1, "读取写入选择"="写入", "holding register values"=u16[] [1], "starting address"=u16 3) -> ()  [unwired: 6 in, 2 out]
        }
        frame #1 {
          # "反控指令"
          # "反控指令\n急停"
          # "3045"
          n243 = Wait (ms)(milliseconds to wait=u32 500 ("等待时间（毫秒）")) -> ()  [unwired: 1 out]
        }
        frame #2 {
          n244 = global write "全局1.vi" "table元素"("反控命令" ("新元素/子数组")) -> ()
          n245 = call "Modbus Master.vi"("Unit ID"=u8 1, "读取写入选择"="写入", "holding register values"=u16[] [0], "starting address"=u16 3) -> ()  [unwired: 6 in, 2 out]
        }
        frame #3 {
        }
      }
    }
    frame "3056" {
      n246 = flat-sequence {
        tunnel: w337 -> [w339]
        frame #0 {
          # "发回给平台"
          # "设置测量时间间隔"
          # "发命令给中控"
          n247 = Search/Split String(string=w339, search string/char (-)="RunInterval" ("搜索字符串/字符(-)")) -> (match + rest of string=w346:string)  [unwired: 1 in, 2 out]
          n248 = Decimal String To Number(string=w346, offset=12 ("偏移量(0)")) -> (number=w342:i32)  [unwired: 1 in, 1 out]
          n249 = Insert Into Array(array=u16[] [] ("holding register values"), index=0 ("索引"), new element=w342) -> (w341:u16[])
          n250 = global write "全局1.vi" "table元素"("反控命令" ("新元素/子数组")) -> ()
          n251 = call "Modbus Master.vi"("Unit ID"=u8 1, "读取写入选择"="写入", "holding register values"=w341, "starting address"=u16 14) -> ()  [unwired: 6 in, 2 out]
        }
        frame #1 {
        }
      }
    }
    frame "3080", "3081", "3082", "3083", "3084", "3085", "3086" {
      n252 = flat-sequence {
        tunnel: w353 -> [w357]
        tunnel: [w355] -> w352
        tunnel: w350 -> [w354]
        tunnel: w352 -> [w382]
        tunnel: [w382] -> w351
        tunnel: w351 -> [w386]
        frame #0 {
          # "30 启动标液核查  1CODmn  2 氨氮  3总磷  4总氮  5CODCr\n31 加标回收\n32 平行样测试\n33 零点核查\n34 跨度核查\n35 校零\n36 校标"
          # "1CODmn  2 氨氮  3总磷  4总氮  5CODCr"
          # "启动单台仪器标液核查"
          # "发命令给中控"
          n253 = Search/Split String(string=w354, search string/char (-)="PolId" ("搜索字符串/字符(-)")) -> (match + rest of string=w362:string)  [unwired: 1 in, 2 out]
          n254 = String Subset(string=w362, offset (0)=6 ("偏移量(0)"), length (rest)=6 ("长度（剩余）")) -> (substring=w359:string)
          n255 = case shown="\"w01019\"" w359 {
            tunnel: [0 ("长度（剩余）") 1 ("长度（剩余）") 2 ("长度（剩余）") 3 ("长度（剩余）") 4 ("长度（剩余）") 5 ("长度（剩余）")] -> w358
            frame "", Default {
            }
            frame "w01019" {
            }
            frame "w21003" {
            }
            frame "w21011" {
            }
            frame "w21001" {
            }
            frame "w01018" {
            }
          }
          n256 = Insert Into Array(array=u16[] [] ("holding register values"), index=0 ("索引"), new element=w358) -> (w363:u16[])
          n257 = case shown="\"3086\"" w357 {
            tunnel: [u16 99 ("starting address") u16 30 ("starting address") u16 31 ("starting address") u16 32 ("starting address") u16 33 ("starting address") u16 34 ("starting address") u16 35 ("starting address") u16 36 ("starting address")] -> w355
            frame "", Default {
            }
            frame "3080" {
            }
            frame "3081" {
            }
            frame "3082" {
            }
            frame "3083" {
            }
            frame "3084" {
            }
            frame "3085" {
            }
            frame "3086" {
            }
          }
          n258 = call "Modbus Master.vi"("Unit ID"=u8 1, "读取写入选择"="写入", "holding register values"=w363, "starting address"=w355) -> ()  [unwired: 6 in, 2 out]
        }
        frame #1 {
          n259 = Wait (ms)(milliseconds to wait=u32 500 ("等待时间（毫秒）")) -> ()  [unwired: 1 out]
        }
        frame #2 {
          n260 = global write "全局1.vi" "table元素"("反控命令" ("新元素/子数组")) -> ()
          n261 = call "Modbus Master.vi"("Unit ID"=u8 1, "读取写入选择"="写入", "holding register values"=u16[] [0], "starting address"=w386) -> ()  [unwired: 6 in, 2 out]
        }
        frame #3 {
        }
      }
    }
  }
